vi "test JSONPath to EXCEL.vi"(11 "Test Case In":refnum<class "Test Config From EXCEL.lvclass">) -> (0 "error out":errorcluster, 3 "Test Case Out":refnum<class "Test Config From EXCEL.lvclass">)   [LabVIEW 2024, in "Test Config From EXCEL.lvclass"]
uses:
  Test Config From EXCEL.lvclass
  C:/Program Files/National Instruments/LabVIEW 2025/vi.lib/Astemes/LUnit/Test Case.lvclass
  <vilib>/Astemes/LUnit/Test Case.lvclass/Test Case.ctl
  Config from EXCEL/Config from EXCEL.lvclass
  <vilib>/Astemes/LUnit/Test Case.lvclass
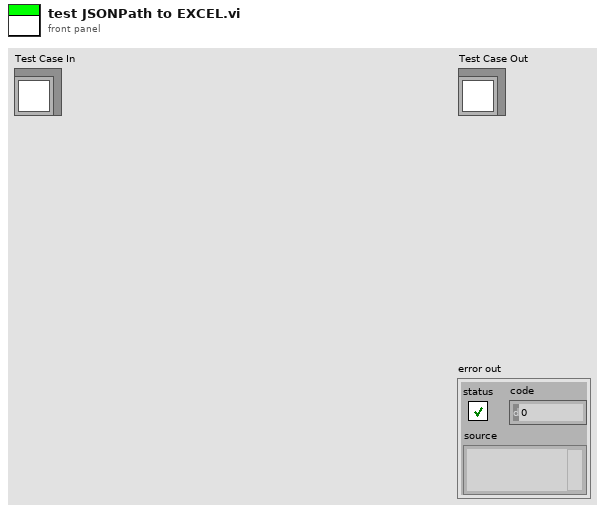
[diagram p1: front panel]
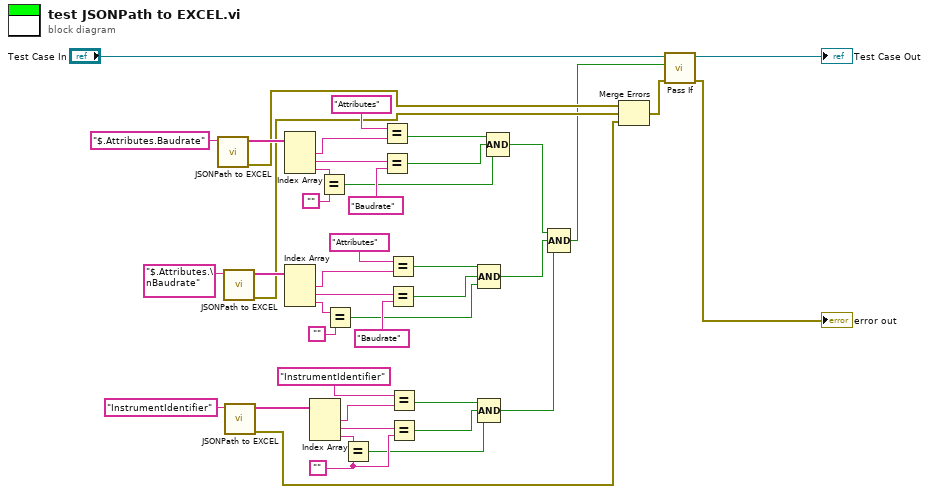
[diagram p0: block diagram]
diagram:
  w24 = ""
  n1 = call "JSONPath to EXCEL.vi"("JSONPath"="$.Attributes.Baudrate") -> ("error out"=w14:errorcluster, "Childs"=w39:string[])  [unwired: 9 in]
  n2 = call "JSONPath to EXCEL.vi"("JSONPath"="$.Attributes.\nBaudrate") -> ("error out"=w13:errorcluster, "Childs"=w29:string[])  [unwired: 9 in]
  n3 = call "JSONPath to EXCEL.vi"("JSONPath"="InstrumentIdentifier") -> ("error out"=w12:errorcluster, "Childs"=w26:string[])  [unwired: 9 in]
  n4 = Index Array(array=w39) -> (element #1=w6:string, element #2=w5:string, element #3=w4:string)  [unwired: 3 in]
  n5 = Index Array(array=w29) -> (element #1=w9:string, element #2=w8:string, element #3=w7:string)  [unwired: 3 in]
  n6 = Index Array(array=w26) -> (element #1=w3:string, element #2=w2:string, element #3=w1:string)  [unwired: 3 in]
  n7 = Equal?(x=w4, y="") -> (x = y?=w33:bool)
  n8 = Equal?(x=w7, y="") -> (x = y?=w21:bool)
  n9 = Equal?(x=w1, y=w24) -> (x = y?=w18:bool)
  n10 = Equal?(x="Attributes", y=w6) -> (x = y?=w35:bool)
  n11 = Equal?(x=w5, y="Baudrate") -> (x = y?=w34:bool)
  n12 = Equal?(x="Attributes", y=w9) -> (x = y?=w23:bool)
  n13 = Equal?(x=w8, y="Baudrate") -> (x = y?=w22:bool)
  n14 = Equal?(x="InstrumentIdentifier", y=w3) -> (x = y?=w20:bool)
  n15 = Equal?(x=w2, y=w24) -> (x = y?=w19:bool)
  n16 = Compound Arithmetic op=AND(w23, w22, w21) -> (w16:bool)
  n17 = Compound Arithmetic op=AND(w20, w19, w18) -> (w15:bool)
  n18 = Compound Arithmetic op=AND(w35, w34, w33) -> (w17:bool)
  n19 = Compound Arithmetic op=AND(w17, w16, w15) -> (w10:bool)
  n20 = Merge Errors(w14, w13, w12) -> (w11:errorcluster)
  n21 = call <vilib>:"Pass If.vi"("error in (no error)"=w11, "Pass?"=w10, "LUnit Test Case In"="Test Case In") -> ("error out"=→"error out":errorcluster, "LUnit Test Case Out"=→"Test Case Out":refnum<class "Test Config From EXCEL.lvclass">)  [unwired: 7 in]
